vi "update.staged.request.vi"(8 "error in":errorcluster, 11 "Promote? (T)":bool=TRUE) -> (0 "error out":errorcluster, 1 "Request":string)   [LabVIEW 2020, in "asset.lvclass"]
uses:
  asset.lvclass
  116a1f63-1174-4f6f-bedf-07de5800daec.vi
  <vilib>/JDP Science/JSONtext/Variant to JSON Text.vi
  <vilib>/JDP Science/JSONtext/LVClass Serializer/JSONtext LVClass Serializer.lvclass
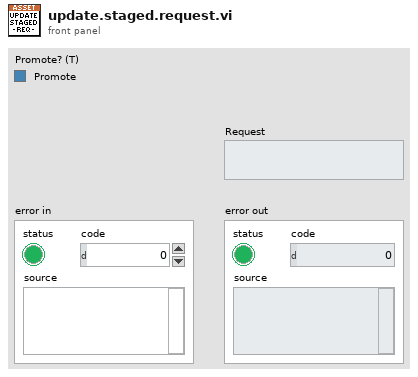
[diagram p1: front panel]
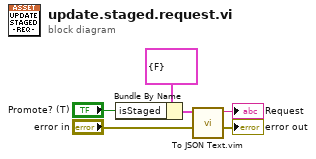
[diagram p0: block diagram]
diagram:
  n1 = Bundle By Name(cluster=cluster{"isStaged":bool} {"isStaged"=FALSE}, "isStaged"="Promote? (T)") -> (w5:cluster{"isStaged":bool})
  n2 = call "To JSON Text.vim"("error in (no error)"="error in", "Anything"=w5) -> ("error out"=→"error out":errorcluster, "<JSON>"=→"Request":string)  [unwired: 8 in]
